vi "1D experiment_v11.vi"() -> ()   [LabVIEW 2010]
uses:
  <vilib>/Utility/inputDevices.llb/closeMouse.vi
  <vilib>/Utility/cursorutil.llb/Set Cursor (Cursor ID).vi
  <vilib>/Utility/inputDevices.llb/mouseAcquire.vi
  User32.dll
panel:
  out "1D Experiment":cluster{"Y":dbl[], "Y":dbl[]}[](graph)
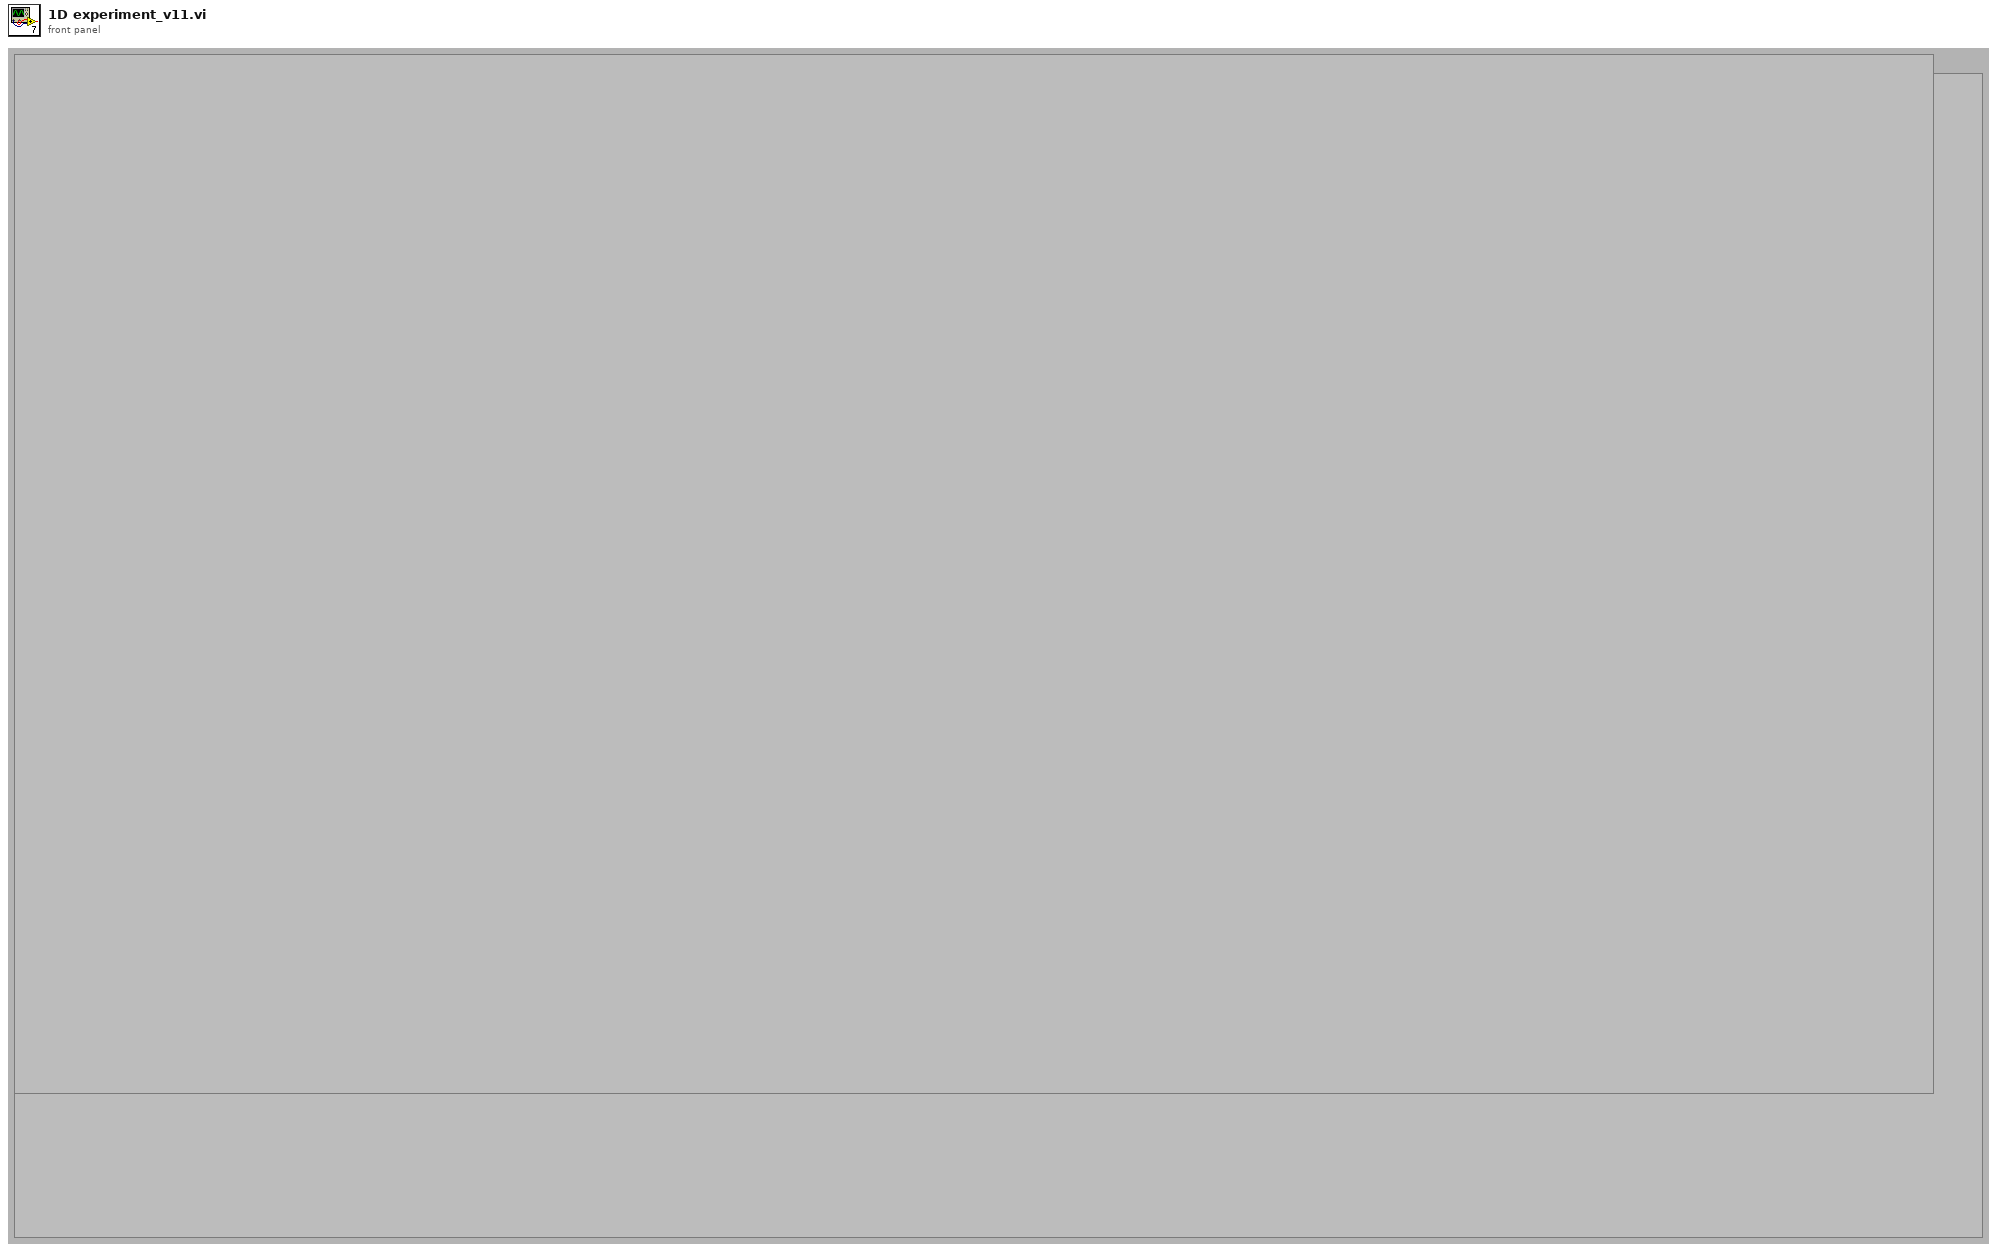
[diagram p1: front panel]
types:
  T1 = cluster{"Radius":dbl, "Center":dbl, "D":dbl, "Valid":bool}
  T2 = typedef "LVAllMonitorsDisplayTypeDef.ctl" = cluster{"Bounds":cluster{"Left":i16, "Top":i16, "Right":i16, "Bottom":i16}, "Depth":i16}[]
  T3 = cluster{"Bounds":cluster{"Left":i16, "Top":i16, "Right":i16, "Bottom":i16}, "Depth":i16}
  T4 = cluster{"Left":i16, "Top":i16, "Right":i16, "Bottom":i16}
  T5 = cluster{"Horizontal":i32, "Vertical":i32, "Scrolling":i32}
  T6 = cluster{"button 1":bool, "button 2":bool, "button 3":bool, "button 4":bool}
  T7 = typedef "LVPoint32TypeDef.ctl" = cluster{"Horizontal":i32, "Vertical":i32}
  T8 = cluster{"Cursor.Cursor Position:Cursor X":dbl, "Cursor.Cursor Position:Cursor X":dbl}
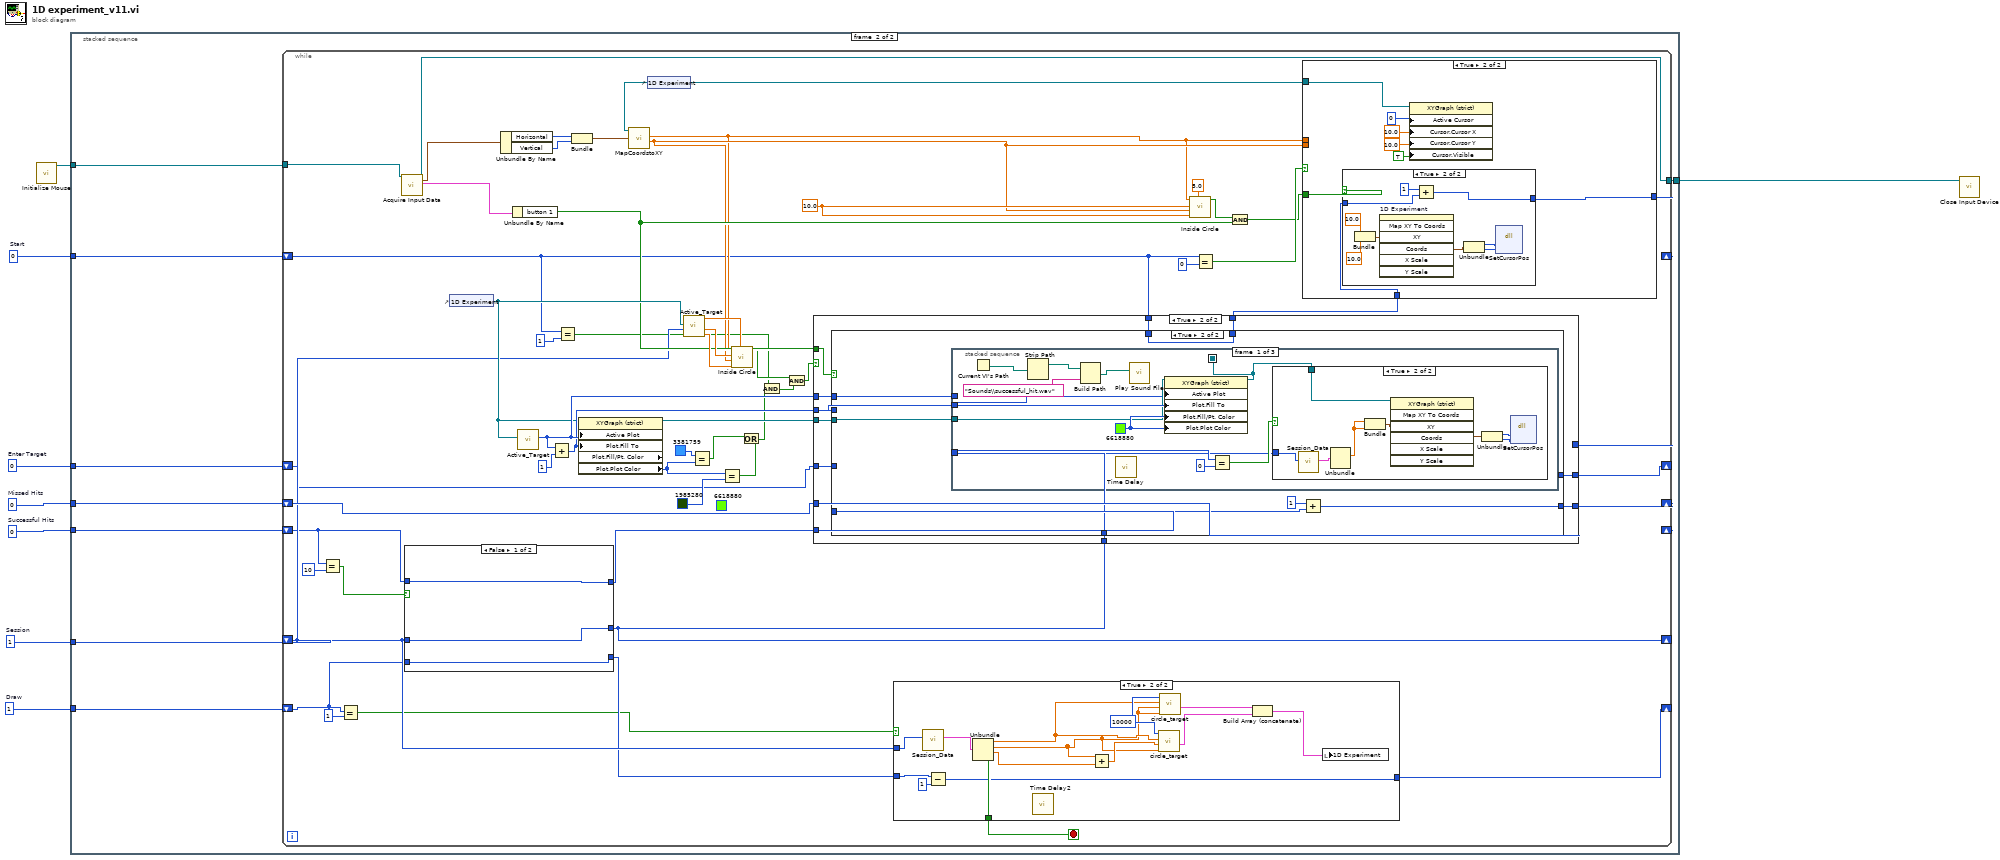
[diagram p0: block diagram]
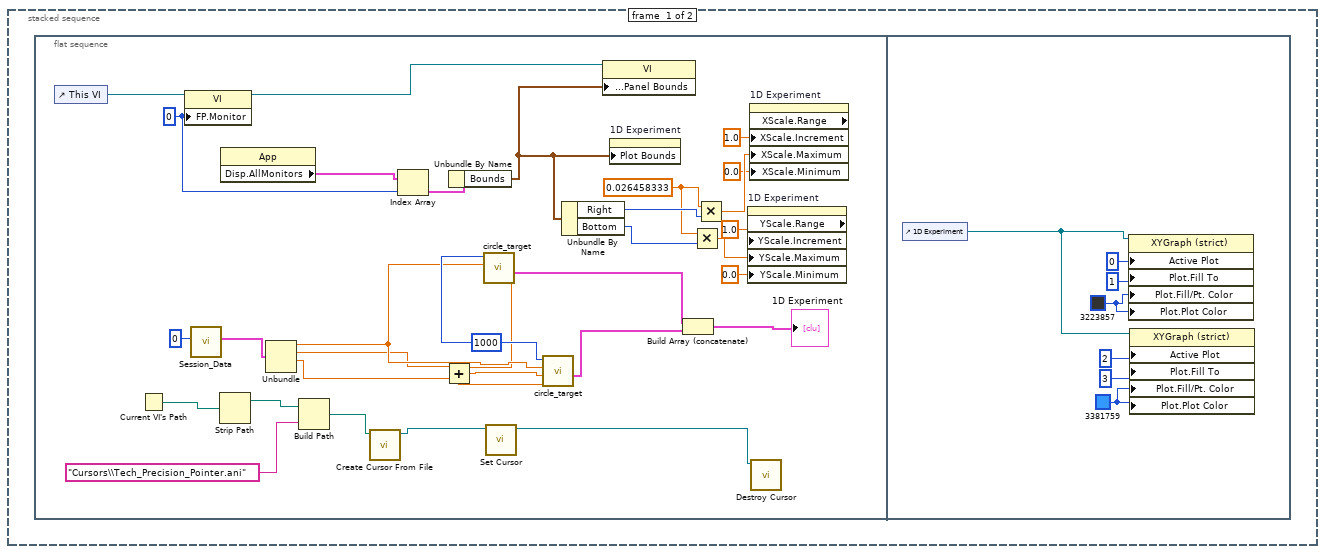
[diagram p2: hidden frame]
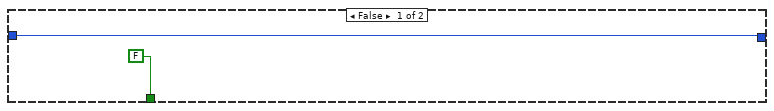
[diagram p3: hidden frame]
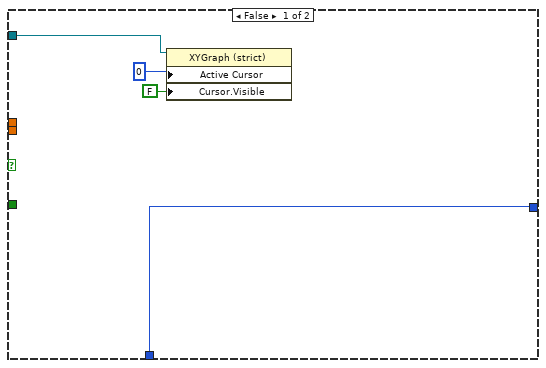
[diagram p4: hidden frame]
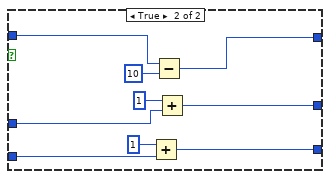
[diagram p6: hidden frame]
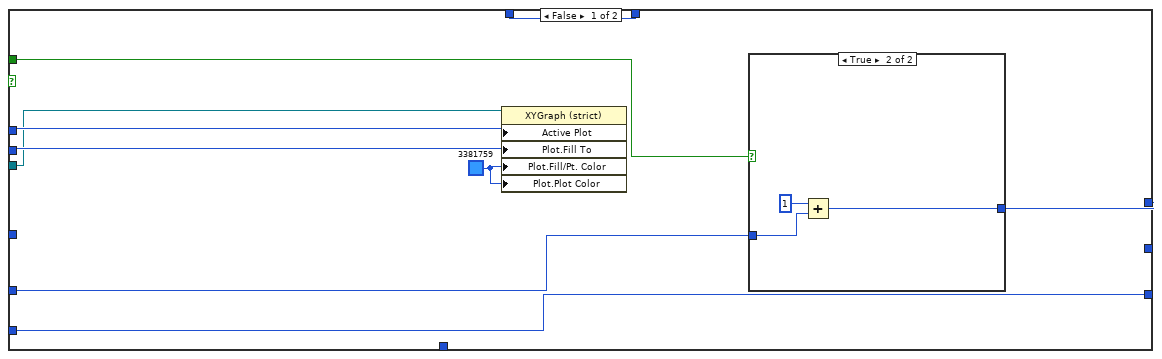
[diagram p7: hidden frame]
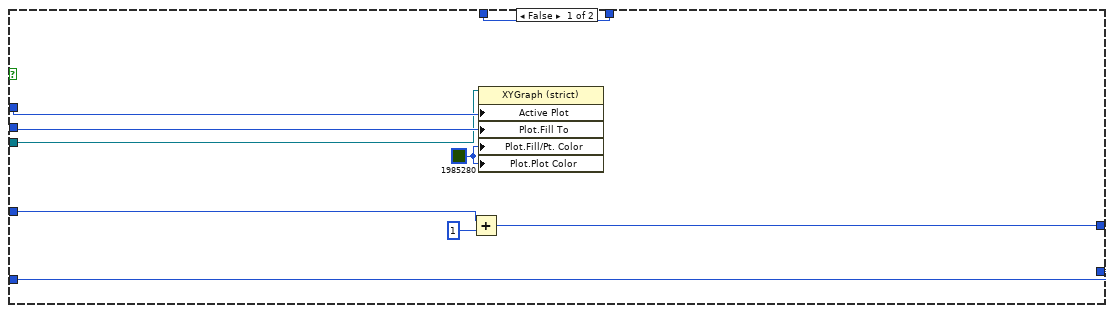
[diagram p9: hidden frame]
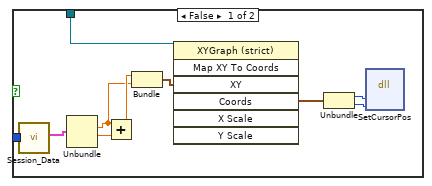
[diagram p10: hidden frame]
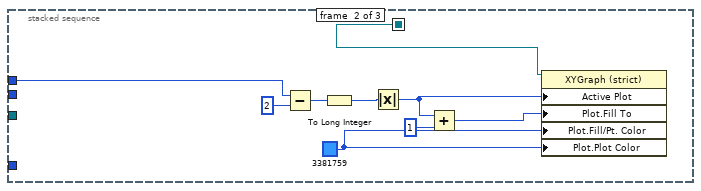
[diagram p11: hidden frame]
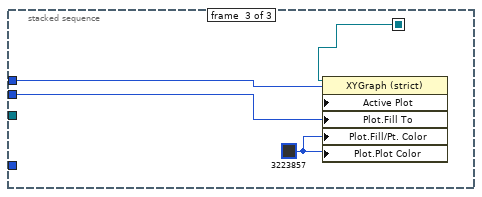
[diagram p12: hidden frame]
diagram:
  w1 = 0  # Enter Target
  w2 = 1  # Draw
  w3 = 0  # Start
  w4 = 1  # Session
  w5 = 0  # Missed Hits
  w6 = 0  # Successful Hits
  n1 = call <vilib>:"Initialize Mouse.vi"() -> ("device ID"=w8:refnum<k1>)  [unwired: 1 in, 10 out]
  n2 = stacked-sequence {
    tunnel: w8 -> [_ w54]
    tunnel: [_ w53] -> w7
    tunnel: w6 -> [_ w52]
    tunnel: w5 -> [_ w51]
    tunnel: w4 -> [_ w50]
    tunnel: w3 -> [_ w49]
    tunnel: w2 -> [_ w48]
    tunnel: w1 -> [_ w47]
    frame #0 {
      n3 = flat-sequence {
        frame #0 {
          w16 = 0.026458333 ("y")
          w27 = u16 0 ("Front Panel Window:Monitor")
          w39 = 1000
          n4 = control-ref of="This VI"() -> (w29:refnum<vi>)
          n5 = Current VI's Path() -> (path=w24:path)
          n6 = property class="VI"(reference=w29, "FP.Monitor"=w27) -> (reference out=w25:refnum<vi>)  [unwired: 1 in, 1 out]
          n7 = call "Session_Data.vi"("Session"=0) -> ("output cluster"=w37:T1)  [unwired: 10 in]
          n8 = Strip Path(path=w24) -> (stripped path=w23:path)  [unwired: 1 out]
          n9 = property class="App"() -> ("Disp.AllMonitors"=w26:T2)  [unwired: 2 in, 2 out]
          n10 = Unbundle(w37) -> ("Radius"=w36:dbl, "Center"=w34:dbl, "D"=w35:dbl)  [unwired: 1 out]
          n11 = Build Path(base path=w23, name or relative path="Cursors\\Tech_Precision_Pointer.ani") -> (appended path=w21:path)
          n12 = call <vilib>:"Create Cursor From File.vi"("cursor file"=w21) -> ("cursor ID"=w20:refnum<k1>)  [unwired: 9 in, 1 out]
          n13 = Index Array(array=w26, index=w27) -> (element=w28:T3)
          n14 = Add(x=w34, y=w35) -> (x+y=w38:dbl)
          n15 = Unbundle By Name(w28) -> ("Bounds"=w18:T4)
          n16 = call "circle_target.vi"("y0"=w34, "x0"=w34, "Radius"=w36, "Pixels"=w39) -> ("Target plots"=w32:cluster{dbl[], dbl[]}[])  [unwired: 7 in]
          n17 = call-poly <vilib>:"Set Cursor.vi"("cursor ID"=w20) -> ("previous cursor ID"=w19:refnum<k1>)  [unwired: 9 in, 1 out]
          n18 = call "circle_target.vi"("y0"=w34, "x0"=w38, "Radius"=w36, "Pixels"=w39) -> ("Target plots"=w33:cluster{dbl[], dbl[]}[])  [unwired: 7 in]
          n19 = Unbundle By Name(w18) -> ("Right"=w17:i16, "Bottom"=w15:i16)
          n20 = property class="VI"(reference=w25, "Front Panel Window:Panel Bounds"=w18) -> ()  [unwired: 1 in, 2 out]
          n21 = property on="1D Experiment" class="XYGraph (strict)"("Plot Bounds"=w18) -> ()  [unwired: 2 in, 2 out]
          n22 = Build Array (concatenate)(w32, w33) -> (→"1D Experiment":cluster{dbl[], dbl[]}[])
          n23 = Multiply(x=w16, y=w15) -> (x*y=w10:dbl)
          n24 = Multiply(x=w16, y=w17) -> (x*y=w13:dbl)
          n25 = property on="1D Experiment" class="XYGraph (strict)" props=["YScale", "Range", "YScale", "Increment", "YScale", "Maximum", "YScale", "Minimum"]("YScale.Increment"=1.0 ("Y Scale.Range:Increment"), "YScale.Maximum"=w10, "YScale.Minimum"=0.0 ("Y Scale.Range:Minimum")) -> ()  [unwired: 2 in, 3 out]
          n26 = property on="1D Experiment" class="XYGraph (strict)" props=["XScale", "Range", "XScale", "Increment", "XScale", "Maximum", "XScale", "Minimum"]("XScale.Increment"=1.0 ("X Scale.Range:Increment"), "XScale.Maximum"=w13, "XScale.Minimum"=0.0 ("X Scale.Range:Minimum")) -> ()  [unwired: 2 in, 3 out]
          n27 = call <vilib>:"Destroy Cursor.vi"("cursor ID"=w19) -> ()  [unwired: 9 in, 1 out]
        }
        frame #1 {
          w45 = u32 3381759
          w42 = u32 3223857
          n28 = control-ref of="1D Experiment"() -> (w46:refnum<vi>)
          n29 = property on="Property Node" class="XYGraph (strict)"(reference=w46, "Active Plot"=u32 0, "Plot.Fill To"=i16 1, "Plot.Fill/Pt. Color"=w42, "Plot.Plot Color"=w42) -> ()  [unwired: 1 in, 2 out]
          n30 = property on="Property Node" class="XYGraph (strict)"(reference=w46, "Active Plot"=u32 2, "Plot.Fill To"=i16 3, "Plot.Fill/Pt. Color"=w45, "Plot.Plot Color"=w45) -> ()  [unwired: 1 in, 2 out]
        }
      }
    }
    frame #1 {
      n31 = while {
        tunnel: w54 -> [w99]
        tunnel: [w98] -> w53
        shift-right: [w94] -> _
        shift-left: w52 -> [w72]
        shift-right: [w92] -> _
        shift-left: w51 -> [w93]
        shift-right: [w64] -> _
        shift-left: w50 -> [w73]
        shift-right: [w78] -> _
        shift-left: w49 -> [w61]
        shift-right: [w69] -> _
        shift-left: w48 -> [w70]
        shift-right: [w65] -> _
        shift-left: w47 -> [w66]
        stop <- w74 stop-if-true
        (unwired) u32 6618880
        w83 = 10.0 ("x0")
        n32 = Equal?(x=w72, y=10) -> (x = y?=w90:bool)
        n33 = Equal?(x=w70, y=1) -> (x = y?=w67:bool)
        n34 = call-poly <vilib>:"Acquire Input Data.vi"("device ID"=w99) -> ("device ID"=w98:refnum<k1>, "axis info"=w97:T5, "button info"=w100:T6)  [unwired: 2 in, 14 out]
        n35 = case shown="False" w90 {
          tunnel: w72 -> [w151 w160]
          tunnel: [w151 w158] -> w89
          tunnel: w73 -> [w150 w157]
          tunnel: [w150 w155] -> w64
          tunnel: w70 -> [w149 w154]
          tunnel: [w149 w152] -> w68
          frame False {
          }
          frame True {
            n36 = Add(x=1, y=w154) -> (x+y=w152:i32)
            n37 = Subtract(x=w160, y=10) -> (x-y=w158:i32)
            n38 = Add(x=1, y=w157) -> (x+y=w155:i32)
          }
        }
        n39 = control-ref of="1D Experiment"() -> (w87:refnum<vi>)
        n40 = Unbundle By Name(w97) -> ("Horizontal"=w96:i32, "Vertical"=w95:i32)
        n41 = Unbundle By Name(w100) -> ("button 1"=w81:bool)
        n42 = call "Active_Target.vi"("XYGraph Refnum"=w87) -> ("Active Plot"=w104:u32)  [unwired: 7 in, 3 out]
        n43 = Add(x=w104, y=u32 1) -> (x+y=w103:u32)
        n44 = Equal?(x=w61, y=1) -> (x = y?=w57:bool)
        n45 = Bundle("Horizontal"=w96, "Vertical"=w95) -> (w84:cluster{"Horizontal":i32, "Vertical":i32})  [unwired: 1 in]
        n46 = property on="Property Node" class="XYGraph (strict)" props=["Active Plot", "Plot", "Fill To", "Plot", "Fill/Pt. Color", "Plot", "Plot Color"](reference=w87, "Active Plot"=w104, "Plot.Fill To"=w103) -> (reference out=w75:refnum<vi>, "Plot.Plot Color"=w77:u32)  [unwired: 1 in, 2 out]
        n47 = control-ref of="1D Experiment"() -> (w55:refnum<vi>)
        n48 = call "MapCoordstoXY.vi"("Coordinates"=w84, "XYGraph Refnum"=w55) -> ("Y(graph)"=w63:dbl, "X (graph)"=w62:dbl)  [unwired: 7 in]
        n49 = call "Active_Target.vi"("Session"=w73, "XYGraph Refnum"=w87) -> ("y0"=w101:dbl, "x0"=w102:dbl, "Radius"=w88:dbl)  [unwired: 6 in, 1 out]
        n50 = Equal?(x=u32 3381759, y=w77) -> (x = y?=w107:bool)
        n51 = Equal?(x=w77, y=u32 1985280) -> (x = y?=w106:bool)
        n52 = call "Inside Circle.vi"("Radius"=w88, "y0"=w101, "y"=w63, "x0"=w102, "x"=w62) -> ("Inside Circle"=w58:bool)  [unwired: 6 in]
        n53 = Or(x=w107, y=w106) -> (x .or. y?=w59:bool)
        n54 = And(x=w57, y=w59) -> (x .and. y?=w56:bool)
        n55 = And(x=w58, y=w56) -> (x .and. y?=w109:bool)
        n56 = case shown="True" w109 {
          tunnel: w81 -> [w167 w185]
          tunnel: w104 -> [w164 w181]
          tunnel: w103 -> [w163 w180]
          tunnel: w89 -> [w168 w184]
          tunnel: [w168 w183] -> w94
          tunnel: w93 -> [w166 w182]
          tunnel: [w165 w182] -> w92
          tunnel: w61 -> [w162 w179]
          tunnel: [w162 w178] -> w76
          tunnel: w75 -> [w161 w177]
          tunnel: w66 -> [_ w176]
          tunnel: [_ w175] -> w65
          tunnel: w64 -> [_ w174]
          frame False {
            w169 = u32 3381759
            n57 = property on="Property Node" class="XYGraph (strict)"(reference=w161, "Active Plot"=w164, "Plot.Fill To"=w163, "Plot.Fill/Pt. Color"=w169, "Plot.Plot Color"=w169) -> ()  [unwired: 1 in, 2 out]
            n58 = case shown="True" w167 {
              tunnel: w166 -> [w170 w173]
              tunnel: [w170 w171] -> w165
              frame False {
              }
              frame True {
                n59 = Add(x=1, y=w173) -> (x+y=w171:i32)
              }
            }
          }
          frame True {
            n60 = case shown="True" w185 {
              tunnel: w184 -> [w193 w202]
              tunnel: [w193 w196] -> w183
              tunnel: w181 -> [w192 w200]
              tunnel: w180 -> [w191 w199]
              tunnel: w179 -> [w190 w198]
              tunnel: [w190 w198] -> w178
              tunnel: w177 -> [w189 w197]
              tunnel: w176 -> [w188 _]
              tunnel: [w186 _] -> w175
              tunnel: w174 -> [_ w195]
              frame False {
                w194 = u32 1985280
                n61 = Add(x=w188, y=1) -> (x+y=w186:i32)
                n62 = property on="Property Node" class="XYGraph (strict)"(reference=w189, "Active Plot"=w192, "Plot.Fill To"=w191, "Plot.Fill/Pt. Color"=w194, "Plot.Plot Color"=w194) -> ()  [unwired: 1 in, 2 out]
              }
              frame True {
                n63 = stacked-sequence {
                  seq-local: [w211 _ _] -> [_ w233 w242]
                  tunnel: w200 -> [w210 w234 w244]
                  tunnel: w199 -> [w213 _ w243]
                  tunnel: w197 -> [w212 _ _]
                  tunnel: w195 -> [w207 _ _]
                  frame #0 {
                    w214 = u32 6618880
                    n64 = Current VI's Path() -> (path=w204:path)
                    n65 = Strip Path(path=w204) -> (stripped path=w203:path)  [unwired: 1 out]
                    n66 = Build Path(base path=w203, name or relative path="Sounds\\successful_hit.wav") -> (appended path=w205:path)
                    n67 = call "Time Delay"() -> ()  [unwired: 11 in, 1 out]
                    n68 = call <vilib>:"Play Sound File.vi"("path"=w205) -> ()  [unwired: 9 in, 2 out]
                    n69 = property on="Property Node" class="XYGraph (strict)"(reference=w212, "Active Plot"=w210, "Plot.Fill To"=w213, "Plot.Fill/Pt. Color"=w214, "Plot.Plot Color"=w214) -> (reference out=w211:refnum<vi>)  [unwired: 1 in, 1 out]
                    n70 = Equal?(x=w210, y=u32 0) -> (x = y?=w208:bool)
                    n71 = case shown="True" w208 {
                      tunnel: w211 -> [w220 w225]
                      tunnel: w207 -> [w217 w229]
                      frame False {
                        n72 = call "Session_Data.vi"("Session"=w217) -> ("output cluster"=w221:T1)  [unwired: 10 in]
                        n73 = Unbundle(w221) -> ("Center"=w215:dbl, "D"=w219:dbl)  [unwired: 2 out]
                        n74 = Add(x=w215, y=w219) -> (x+y=w216:dbl)
                        n75 = Bundle(w216, "Center"=w215) -> (w218:cluster{dbl, "Center":dbl})  [unwired: 1 in]
                        n76 = invoke on="Invoke Node" class="XYGraph (strict)" method="Map XY To Coords"(reference=w220, "XY"=w218) -> ("Coords"=w224:T7)  [unwired: 5 in, 6 out]
                        n77 = Unbundle(w224) -> ("Horizontal"=w223:i32, "Vertical"=w222:i32)
                        n78 = dll-call lib="User32.dll" fn="SetCursorPos"(w223, w222) -> ()  [unwired: 6 in, 2 out]
                      }
                      frame True {
                        n79 = call "Session_Data.vi"("Session"=w229) -> ("output cluster"=w228:T1)  [unwired: 10 in]
                        n80 = Unbundle(w228) -> ("Center"=w227:dbl)  [unwired: 3 out]
                        n81 = Bundle("Center"=w227, "Center"=w227) -> (w226:cluster{"Center":dbl, "Center":dbl})  [unwired: 1 in]
                        n82 = invoke on="Invoke Node" class="XYGraph (strict)" method="Map XY To Coords"(reference=w225, "XY"=w226) -> ("Coords"=w232:T7)  [unwired: 5 in, 6 out]
                        n83 = Unbundle(w232) -> ("Horizontal"=w231:i32, "Vertical"=w230:i32)
                        n84 = dll-call lib="User32.dll" fn="SetCursorPos"(w231, w230) -> ()  [unwired: 6 in, 2 out]
                      }
                    }
                  }
                  frame #1 {
                    w241 = u32 3381759
                    n85 = Subtract(x=w234, y=u32 2) -> (x-y=w238:u32)
                    n86 = To Long Integer(number=w238) -> (32bit integer=w237:i32)
                    n87 = Absolute Value(x=w237) -> (abs(x)=w235:i32)
                    n88 = Add(x=w235, y=u32 1) -> (x+y=w239:u32)
                    n89 = property on="Property Node" class="XYGraph (strict)"(reference=w233, "Active Plot"=w235, "Plot.Fill To"=w239, "Plot.Fill/Pt. Color"=w241, "Plot.Plot Color"=w241) -> ()  [unwired: 1 in, 2 out]
                  }
                  frame #2 {
                    w245 = u32 3223857
                    n90 = property on="Property Node" class="XYGraph (strict)"(reference=w242, "Active Plot"=w244, "Plot.Fill To"=w243, "Plot.Fill/Pt. Color"=w245, "Plot.Plot Color"=w245) -> ()  [unwired: 1 in, 2 out]
                  }
                }
                n91 = Add(x=1, y=w202) -> (x+y=w196:i32)
              }
            }
          }
        }
        n92 = case shown="True" w67 {
          tunnel: [FALSE ("Valid") w118] -> w74
          tunnel: w73 -> [_ w117]
          tunnel: [w111 w115] -> w69
          tunnel: w68 -> [w111 w114]
          frame False {
          }
          frame True {
            w126 = 10000
            n93 = call "Session_Data.vi"("Session"=w117) -> ("output cluster"=w124:T1)  [unwired: 10 in]
            n94 = Subtract(x=w114, y=1) -> (x-y=w115:i32)
            n95 = Unbundle(w124) -> ("Radius"=w123:dbl, "Center"=w121:dbl, "D"=w122:dbl, "Valid"=w118:bool)
            n96 = call "Time Delay2"() -> ()  [unwired: 11 in, 1 out]
            n97 = Add(x=w121, y=w122) -> (x+y=w125:dbl)
            n98 = call "circle_target.vi"("y0"=w121, "x0"=w125, "Radius"=w123, "Pixels"=w126) -> ("Target plots"=w119:cluster{dbl[], dbl[]}[])  [unwired: 7 in]
            n99 = call "circle_target.vi"("y0"=w121, "x0"=w121, "Radius"=w123, "Pixels"=w126) -> ("Target plots"=w120:cluster{dbl[], dbl[]}[])  [unwired: 7 in]
            n100 = Build Array (concatenate)(w120, w119) -> (w113:cluster{dbl[], dbl[]}[])
            n101 = local write "1D Experiment"(w113) -> ()
          }
        }
        n102 = call "Inside Circle.vi"("Radius"=5.0, "y0"=w83, "y"=w63, "x0"=w83, "x"=w62) -> ("Inside Circle"=w80:bool)  [unwired: 6 in]
        n103 = Equal?(x=w61, y=0) -> (x = y?=w85:bool)
        n104 = And(x=w80, y=w81) -> (x .and. y?=w79:bool)
        n105 = case shown="True" w85 {
          tunnel: w55 -> [w127 w132]
          tunnel: w62 -> [_ _]
          tunnel: w63 -> [_ _]
          tunnel: w79 -> [_ w135]
          tunnel: w76 -> [w130 w134]
          tunnel: [w130 w133] -> w78
          frame False {
            n106 = property on="Property Node" class="XYGraph (strict)"(reference=w127, "Active Cursor"=u32 0, "Cursor.Visible"=FALSE) -> ()  [unwired: 1 in, 2 out]
          }
          frame True {
            n107 = case shown="True" w135 {
              tunnel: w134 -> [w139 w148]
              tunnel: [w139 w146] -> w133
              frame False {
              }
              frame True {
                n108 = Bundle("Cursor.Cursor Position:Cursor X"=10.0, "Cursor.Cursor Position:Cursor X"=10.0) -> (w143:T8)  [unwired: 1 in]
                n109 = invoke on="1D Experiment" class="XYGraph (strict)" method="Map XY To Coords"("XY"=w143) -> ("Coords"=w142:T7)  [unwired: 6 in, 6 out]
                n110 = Add(x=1, y=w148) -> (x+y=w146:i32)
                n111 = Unbundle(w142) -> ("Horizontal"=w141:i32, "Vertical"=w140:i32)
                n112 = dll-call lib="User32.dll" fn="SetCursorPos"(w141, w140) -> ()  [unwired: 6 in, 2 out]
              }
            }
            n113 = property on="Property Node" class="XYGraph (strict)"(reference=w132, "Active Cursor"=u32 0, "Cursor.Cursor X"=10.0 ("Cursor.Cursor Position:Cursor X"), "Cursor.Cursor Y"=10.0 ("Cursor.Cursor Position:Cursor Y"), "Cursor.Visible"=TRUE) -> ()  [unwired: 1 in, 2 out]
          }
        }
      }
    }
  }
  n114 = call-poly <vilib>:"Close Input Device.vi"("device ID"=w7) -> ()  [unwired: 1 in, 9 out]
